vi "save_file.vi"(8 "error in (no error)":errorcluster, 11 "program states  in":T1=enum."espresso") -> (0 "error out":errorcluster, 3 "program states out":T1)   [LabVIEW 2024]
doc: "Writes date and type of coffe made to xml file."
uses:
  Controls/#typedef_program_states_kawa.ctl
  <vilib>/Utility/file.llb/Write Delimited Spreadsheet (string).vi
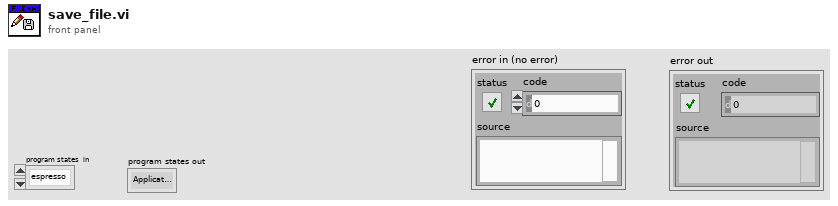
[diagram p1: front panel]
types:
  T1 = typedef "#typedef_program_states_kawa.ctl" = enum16{"Application Error", "init", "idle", "espresso", "espresso macchiato", "caffe latte", "cafe mocha", "stop"}
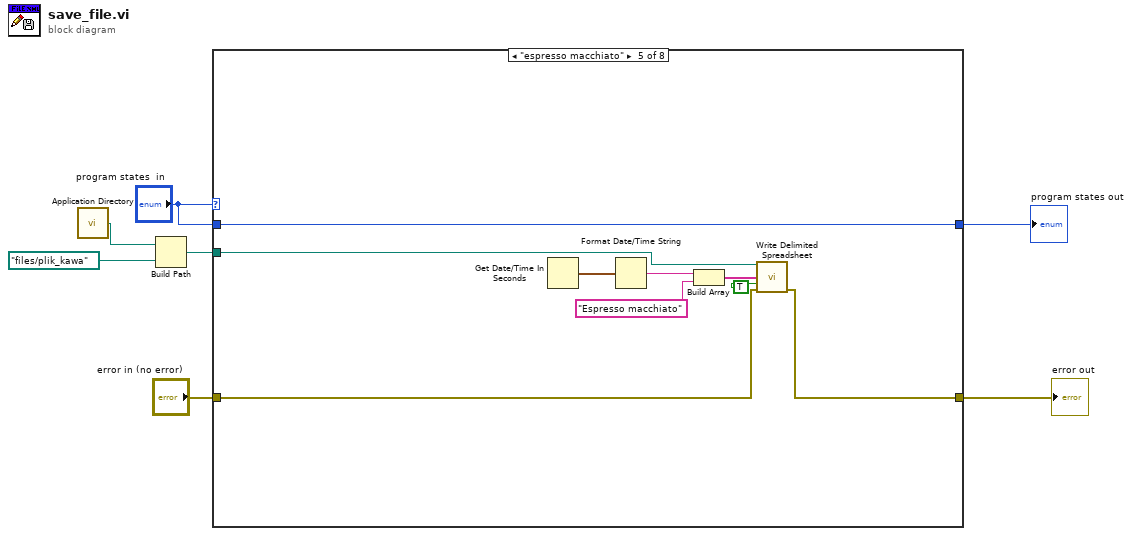
[diagram p0: block diagram]
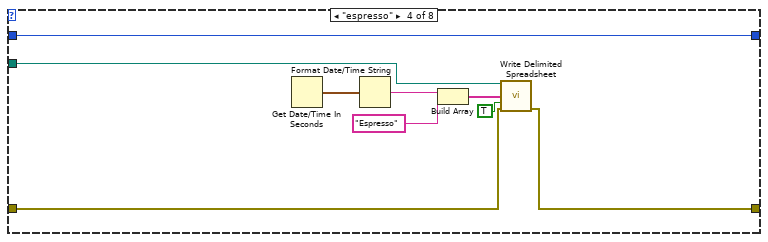
[diagram p5: hidden frame]
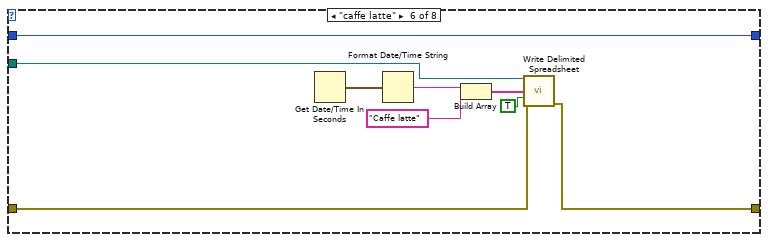
[diagram p6: hidden frame]
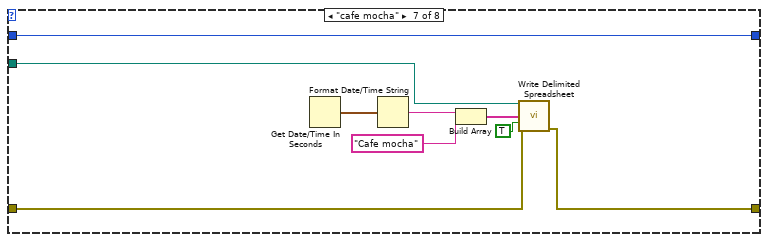
[diagram p7: hidden frame]
diagram:
  n1 = call <vilib>:"Application Directory.vi"() -> ("Application Directory"=w3:path)
  n2 = Build Path(base path=w3, name or relative path=path "files/plik_kawa" ("file path (dialog if empty)")) -> (appended path=w1:path)
  n3 = case shown="\"espresso macchiato\"" "program states  in" {
    tunnel: [w8 w11 w12 w22 w31 w40 w49 w50] -> w7
    tunnel: "error in (no error)" -> [w9 w10 w13 w16 w25 w33 w42 w51]
    tunnel: [w9 w10 w13 w15 w24 w34 w43 w51] -> w5
    tunnel: "program states  in" -> [w8 w11 w12 w22 w31 w40 w49 w50]
    tunnel: w1 -> [_ _ _ w14 w23 w32 w41 _]
    frame "Application Error", Default {
    }
    frame "init" {
    }
    frame "idle" {
    }
    frame "espresso" {
      n4 = Get Date/Time In Seconds() -> (seconds since 1Jan1904=w20:timestamp)
      n5 = Format Date/Time String(seconds (now)=w20) -> (date/time string=w19:string)  [unwired: 2 in]
      n6 = Build Array(w19, "Espresso" ("text")) -> (w18:string[])
      n7 = call-poly <vilib>:"Write Delimited Spreadsheet.vi"("file path (dialog if empty)"=w14, "1D data"=w18, "append to file? (new file:F)"=TRUE, "error in (no error)"=w16) -> ("error out"=w15:errorcluster)  [unwired: 10 in, 1 out]
    }
    frame "espresso macchiato" {
      n8 = Get Date/Time In Seconds() -> (seconds since 1Jan1904=w30:timestamp)
      n9 = Format Date/Time String(seconds (now)=w30) -> (date/time string=w29:string)  [unwired: 2 in]
      n10 = Build Array(w29, "Espresso macchiato" ("text")) -> (w28:string[])
      n11 = call-poly <vilib>:"Write Delimited Spreadsheet.vi"("file path (dialog if empty)"=w23, "1D data"=w28, "append to file? (new file:F)"=TRUE, "error in (no error)"=w25) -> ("error out"=w24:errorcluster)  [unwired: 10 in, 1 out]
    }
    frame "caffe latte" {
      n12 = Get Date/Time In Seconds() -> (seconds since 1Jan1904=w38:timestamp)
      n13 = Format Date/Time String(seconds (now)=w38) -> (date/time string=w37:string)  [unwired: 2 in]
      n14 = Build Array(w37, "Caffe latte" ("text")) -> (w36:string[])
      n15 = call-poly <vilib>:"Write Delimited Spreadsheet.vi"("file path (dialog if empty)"=w32, "1D data"=w36, "append to file? (new file:F)"=TRUE, "error in (no error)"=w33) -> ("error out"=w34:errorcluster)  [unwired: 10 in, 1 out]
    }
    frame "cafe mocha" {
      n16 = Get Date/Time In Seconds() -> (seconds since 1Jan1904=w47:timestamp)
      n17 = Format Date/Time String(seconds (now)=w47) -> (date/time string=w46:string)  [unwired: 2 in]
      n18 = Build Array(w46, "Cafe mocha" ("text")) -> (w45:string[])
      n19 = call-poly <vilib>:"Write Delimited Spreadsheet.vi"("file path (dialog if empty)"=w41, "1D data"=w45, "append to file? (new file:F)"=TRUE, "error in (no error)"=w42) -> ("error out"=w43:errorcluster)  [unwired: 10 in, 1 out]
    }
    frame "stop" {
    }
  }
  "program states out" <- w7
  "error out" <- w5
